vi "test - Basic Function.vi"(8 "error in (no error)":errorcluster, 11 "TestCase in":refnum<class "testcase-Broadcast Registry.lvclass">) -> (0 "error out":errorcluster, 3 "TestCase out":refnum<class "testcase-Broadcast Registry.lvclass">)   [LabVIEW 2017, in "testcase-Broadcast Registry.lvclass"]
uses:
  testcase-Broadcast Registry.lvclass
  f1ab6f25-c30d-499f-96ca-3a55fa643449.vi
  src/user.lib/_NEVSTOP/Communicable State Machine(CSM)/AdvanceAPI/CSM - Revert Arguments-Safe String.vi
  src/user.lib/_NEVSTOP/Communicable State Machine(CSM)/_Shared/Trim Single-line Text.vi
  src/user.lib/_NEVSTOP/Communicable State Machine(CSM)/AdvanceAPI/CSM - Make String Arguments Safe.vi
  src/user.lib/_NEVSTOP/Communicable State Machine(CSM)/AdvanceAPI/CSM - Break Down Multiple States String.vi
  src/user.lib/_NEVSTOP/Communicable State Machine(CSM)/AdvanceAPI/CSM - Compact Multiple States.vi
  src/user.lib/_NEVSTOP/Communicable State Machine(CSM)/AdvanceAPI/CSM - Keywords.vi
  <vilib>/addons/_JKI Toolkits/VI Tester/TestCase.llb/TestCase.lvclass
  src/user.lib/_NEVSTOP/Communicable State Machine(CSM)/Communicable State Machine.lvlib
  C:/Program Files (x86)/National Instruments/LabVIEW 2017/vi.lib/addons/_JKI Toolkits/VI Tester/TestCase.llb/TestCase.lvclass
panel:
  out "Error Occurred":errorcluster
  out "State History":string
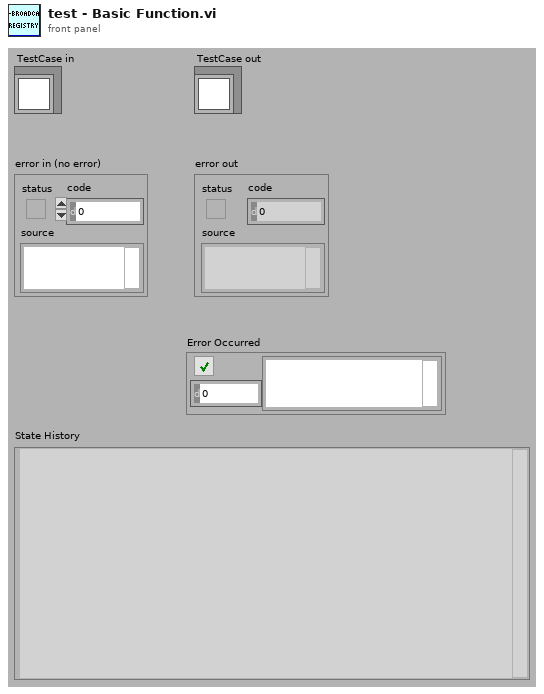
[diagram p1: front panel]
types:
  T1 = enum32{"Invalid", "Standard", "Closed", "Hidden", "Minimized", "Maximized"}
  T2 = enum32{"invalid app kind", "Development System", "Run Time System", "Student Edition", "Embedded LabVIEW", "Evaluation", "Custom"}
  T3 = cluster{"Status":string, "Source CSM":string, "Target CSM":string, "Target API":string}[]
  T4 = typedef "Communicable State Machine.lvlib/_CSM_Response Source Message.ctl" = cluster{"‘State":string, "’Arguments":string, "’Error":errorcluster}
  T5 = cluster{"Current VI Reference":refnum<vi>, "Close Panel on Exit?":bool}
  T6 = cluster{"Core":cluster{"Current VI Reference":refnum<vi>, "Close Panel on Exit?":bool}, "Your Boolean data":bool, "Your string data":string}
  T7 = cluster{"Status":string, "Source CSM":string, "Target CSM":string, "Target API":string}
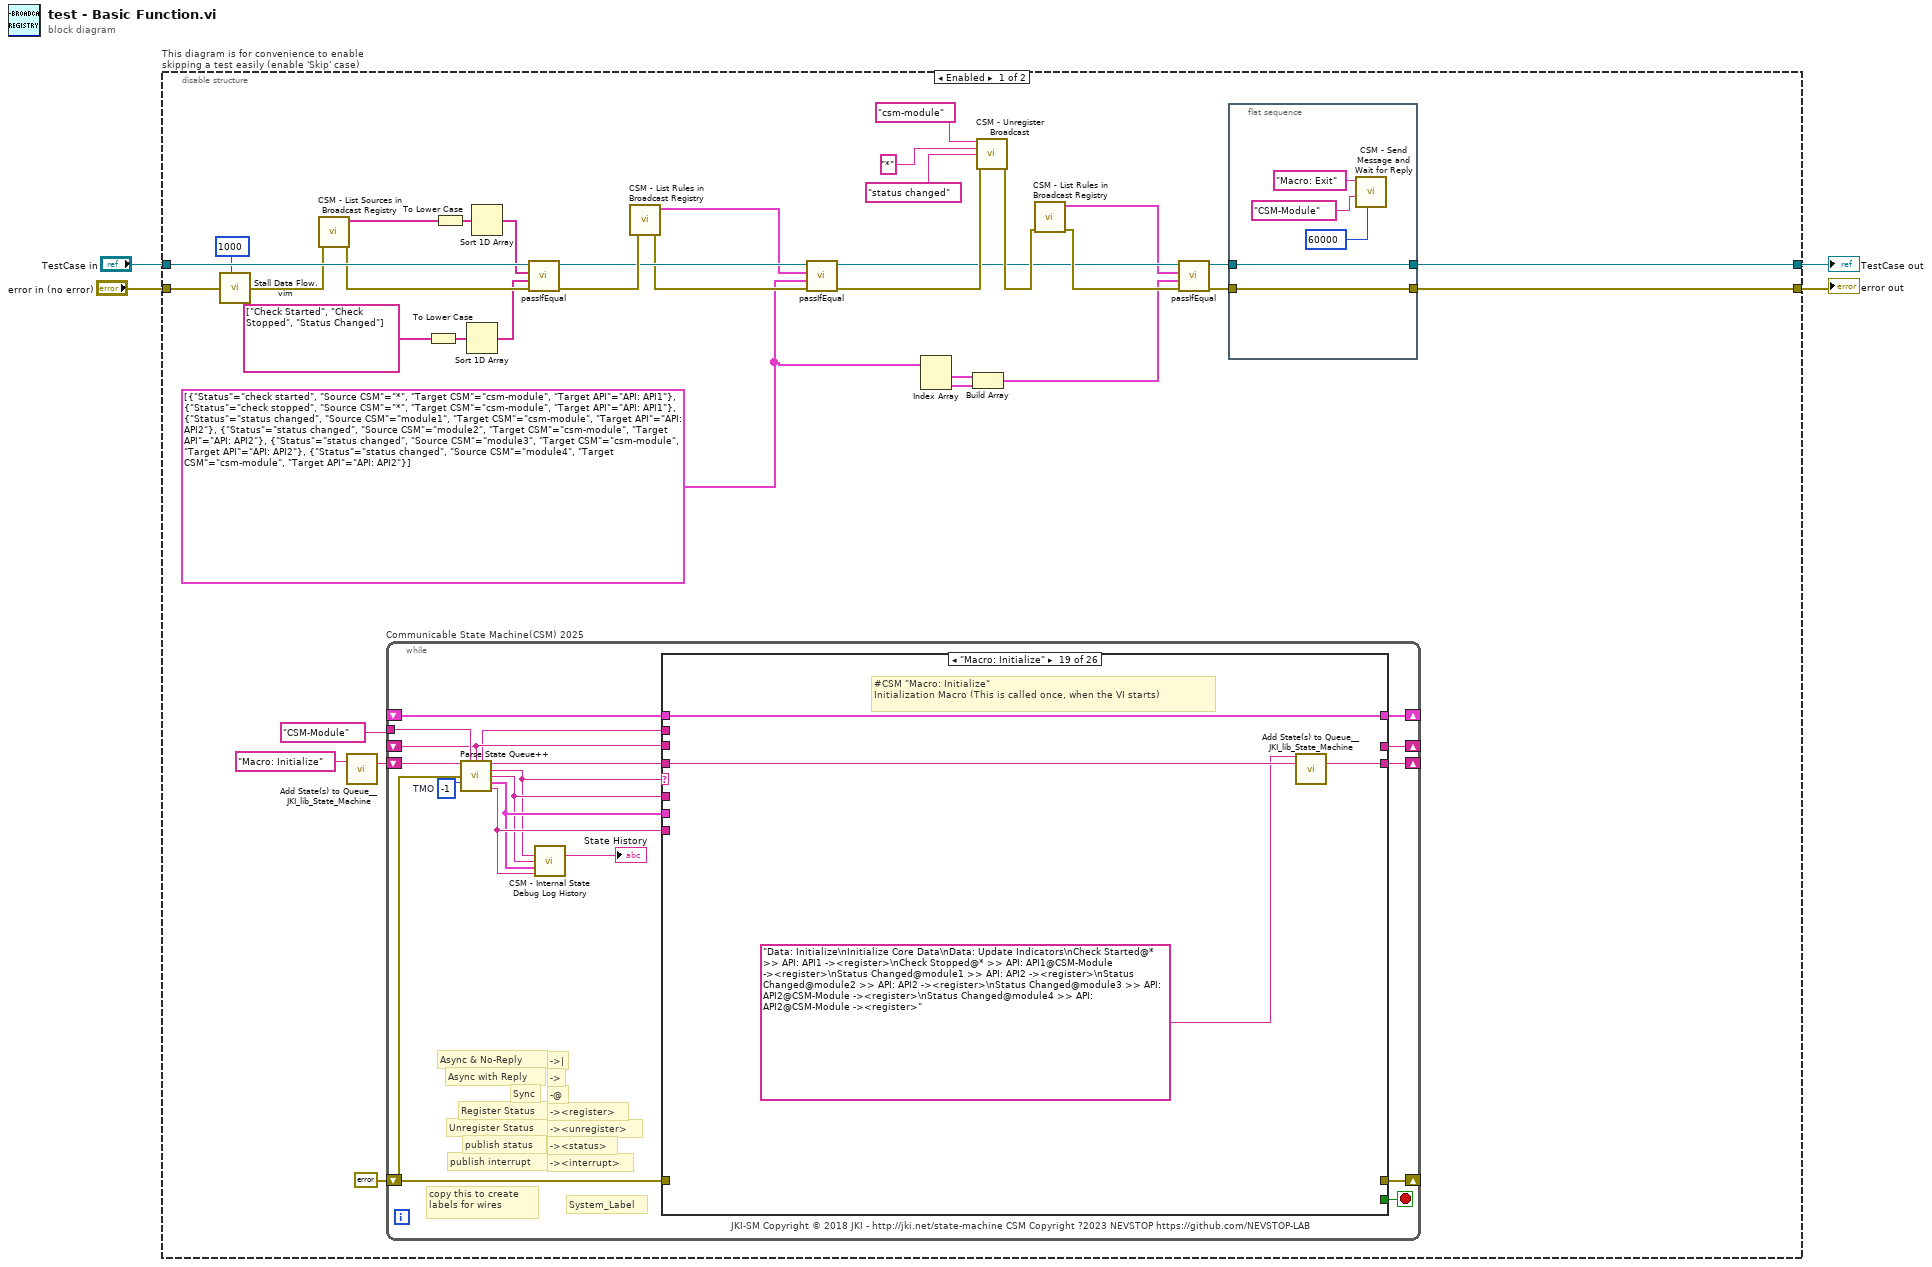
[diagram p0: block diagram]
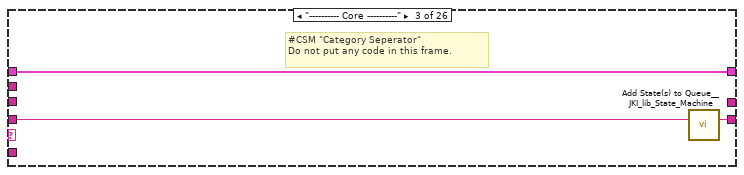
[diagram p4: hidden frame]
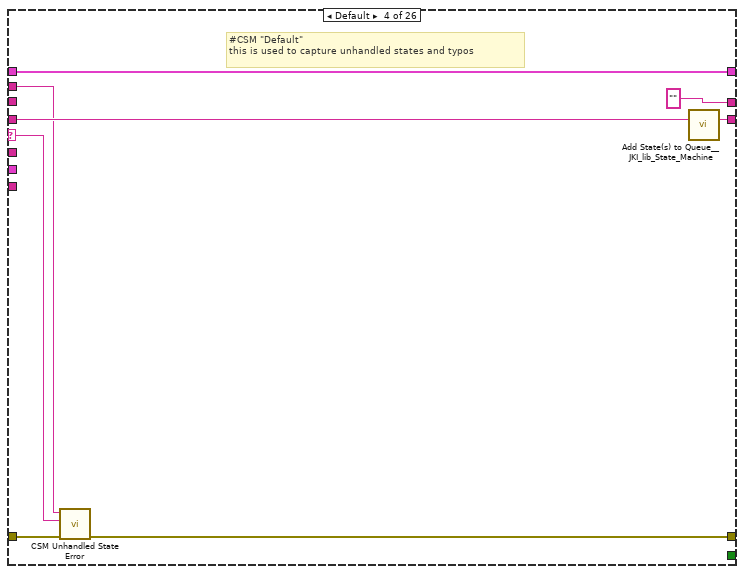
[diagram p5: hidden frame]
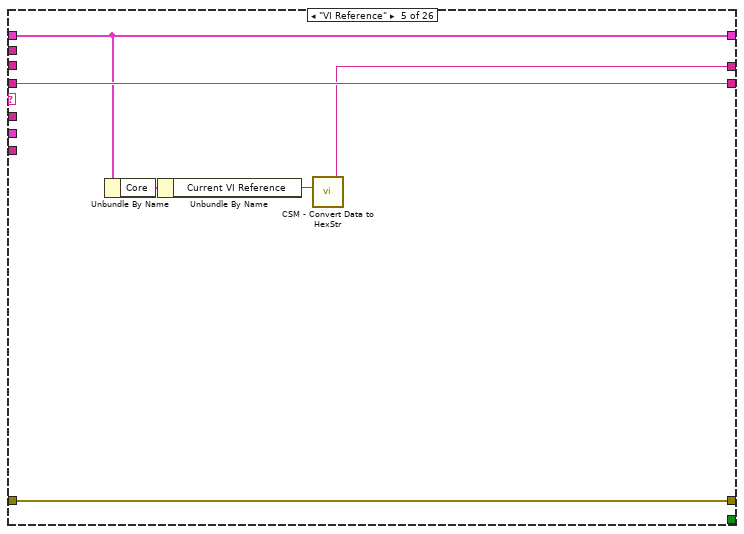
[diagram p6: hidden frame]
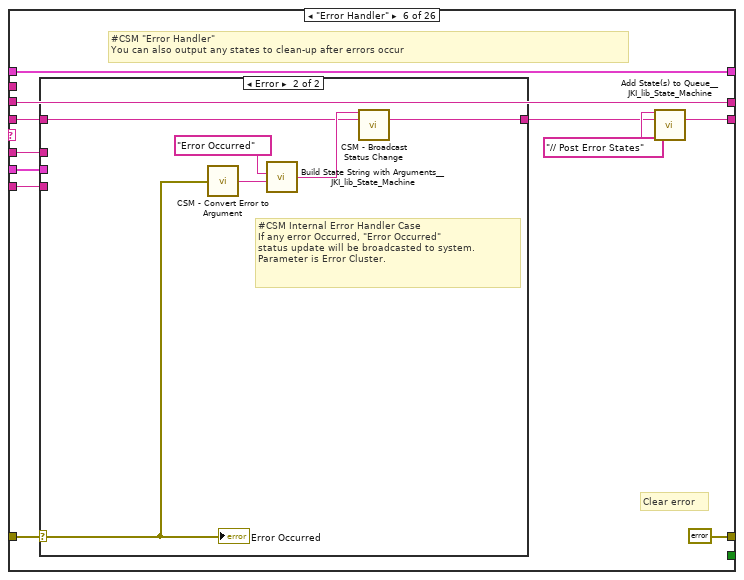
[diagram p7: hidden frame]
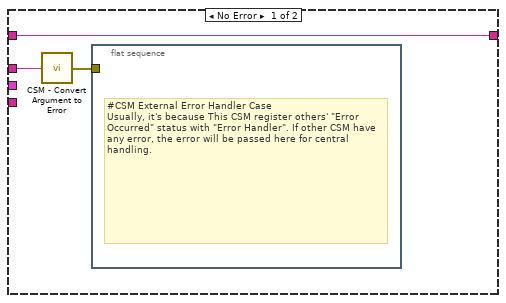
[diagram p8: hidden frame]
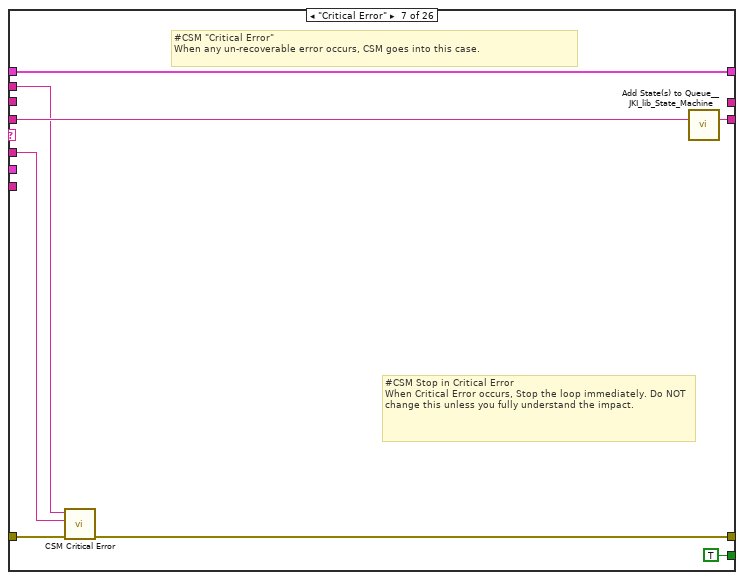
[diagram p9: hidden frame]
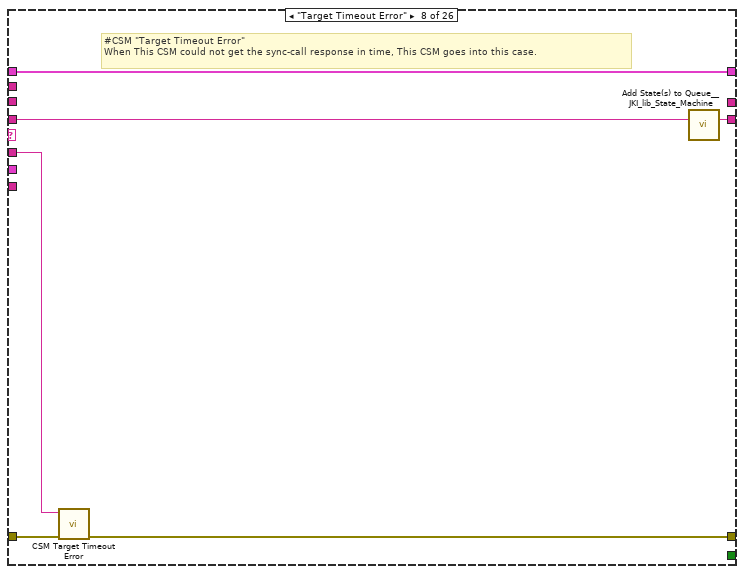
[diagram p10: hidden frame]
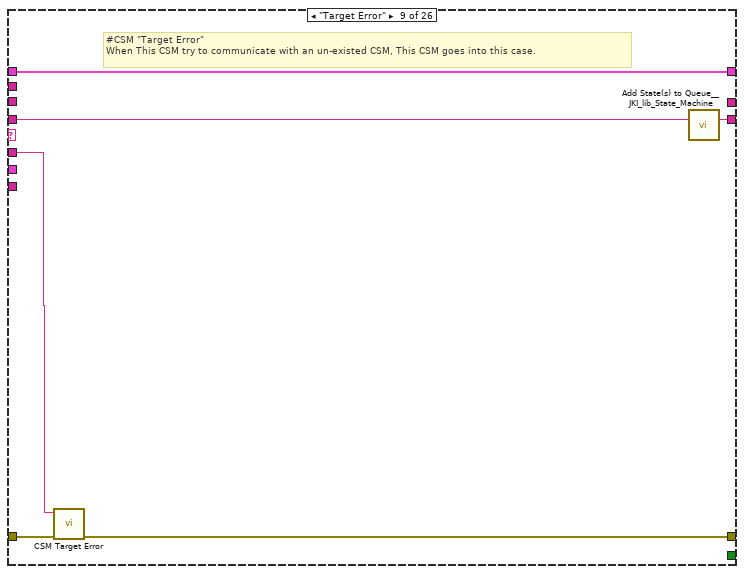
[diagram p11: hidden frame]
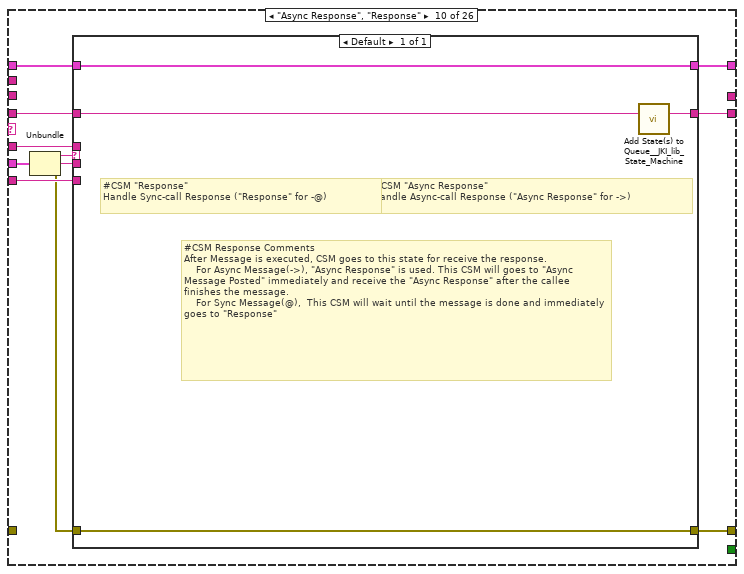
[diagram p12: hidden frame]
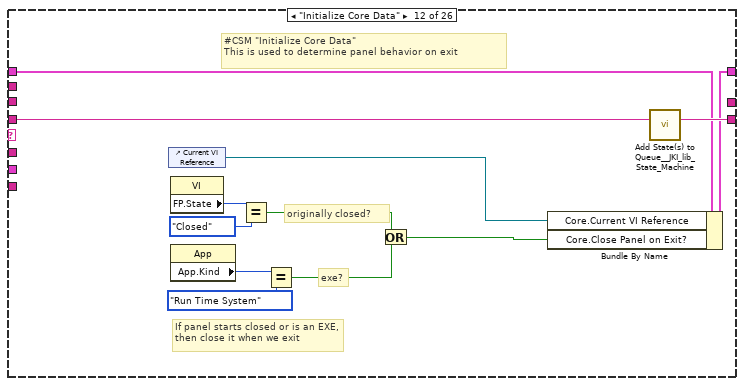
[diagram p14: hidden frame]
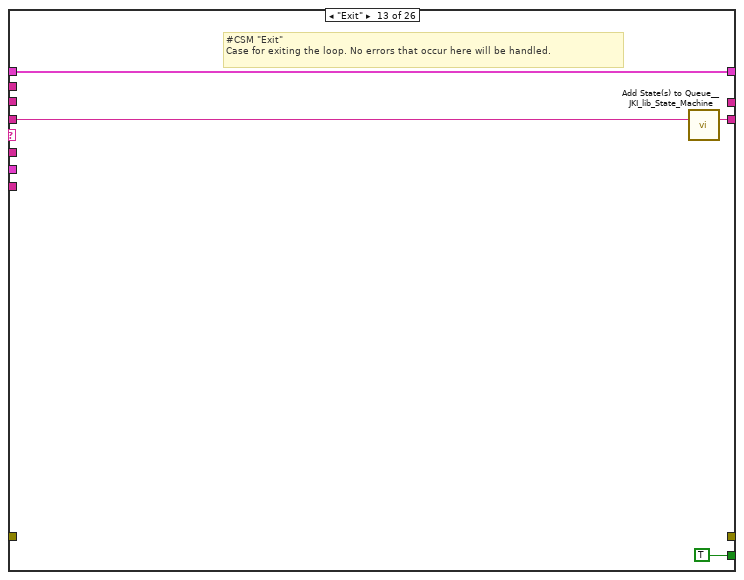
[diagram p15: hidden frame]
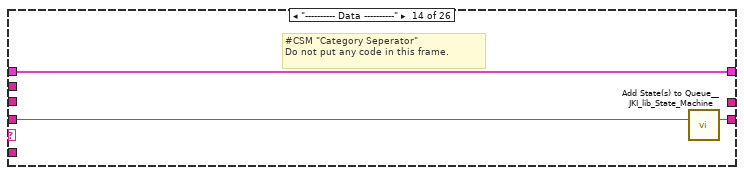
[diagram p16: hidden frame]
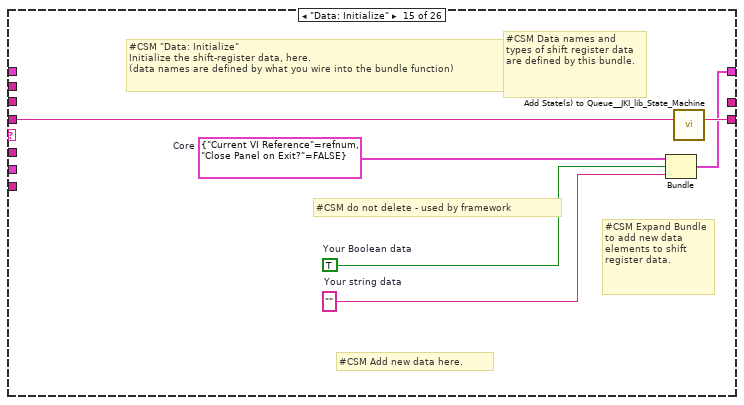
[diagram p17: hidden frame]
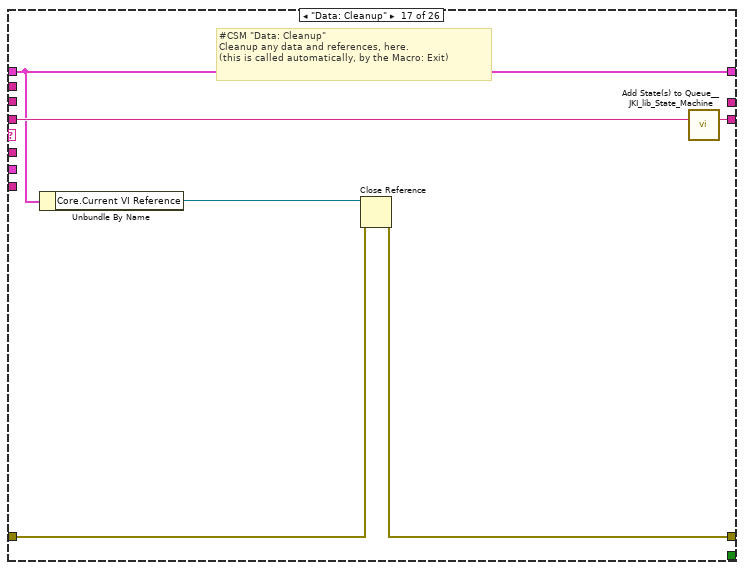
[diagram p19: hidden frame]
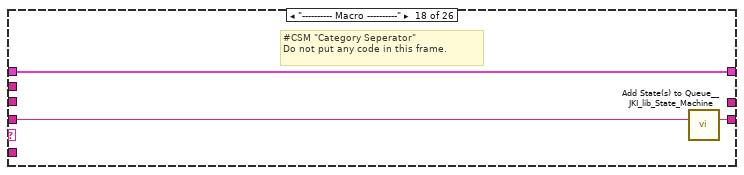
[diagram p20: hidden frame]
diagram:
  n1 = disable-structure "This diagram is for convenience to enable skipping a test easily (enable 'Skip' case)" shown="Enabled" {
    disable-tunnel: "TestCase in" -> [w39 w210]
    disable-tunnel: [w21 w208] -> w1
    disable-tunnel: [w28 w209] -> w3
    disable-tunnel: "error in (no error)" -> [w38 w207]
    frame Enabled {
      w8 = T3 [{"Status"="check started", "Source CSM"="*", "Target CSM"="csm-module", "Target API"="API: API1"}, {"Status"="check stopped", "Source CSM"="*", "Target CSM"="csm-module", "Target API"="API: API1"}, {"Status"="status changed", "Source CSM"="module1", "Target CSM"="csm-module", "Target API"="API: API2"}, {"Status"="status changed", "Source CSM"="module2", "Target CSM"="csm-module", "Target API"="API: API2"}, {"Status"="status changed", "Source CSM"="module3", "Target CSM"="csm-module", "Target API"="API: API2"}, {"Status"="status changed", "Source CSM"="module4", "Target CSM"="csm-module", "Target API"="API: API2"}] ("Entries")
      n2 = call "Stall Data Flow.vim"("value in"=w38, "milliseconds to wait"=u32 1000) -> ("value out"=w33:errorcluster)  [unwired: 1 out]
      n3 = call "CSM - List Sources in Broadcast Registry.vi"("error in (no error)"=w33) -> ("error out"=w31:errorcluster, "Broadcast Names"=w30:string[])  [unwired: 9 in]
      n4 = call <vilib>:"Add State(s) to Queue__JKI_lib_State_Machine.vi"("State(s) in (\"\")"="Macro: Initialize" ("Init State(\"Macro: Initialize\")")) -> ("States Out"=w37:string)  [unwired: 14 in]
      n5 = while "Communicable State Machine(CSM) 2025" {
        shift-right: [w57] -> _
        shift-left: _ -> [w56]
        shift-right: [w60] -> _
        shift-left: errorcluster {"status"=FALSE, "code"=0, "source"=""} ("error out") -> [w46]
        shift-right: [w59] -> _
        shift-left: w37 -> [w61]
        tunnel: "CSM-Module" ("Name (\"\" to Use UUID)") -> [w53]
        shift-right: [w54] -> _
        shift-left: _ -> [w48]
        stop <- w58 stop-if-true
        w55 = -1  # TMO
        # "-><interrupt>"
        # "-><status>"
        # "-><unregister>"
        # "-><register>"
        # "-@"
        # "->"
        # "->|"
        # "publish interrupt"
        # "publish status"
        # "Unregister Status"
        # "Register Status"
        # "Sync"
        # "Async with Reply"
        # "Async & No-Reply"
        # "JKI-SM Copyright © 2018 JKI - http://jki.net/state-machine CSM Copyright ?2023 NEVSTOP https://github.com/NEVSTOP-LAB"
        # "copy this to create labels for wires"
        # "System_Label"
        n6 = call "Parse State Queue++.vi"("State Queue"=w61, "Name (\"\" to Use UUID)"=w53, "Response Arguments"=w48, "Previous Error"=w46, "Dequeue (1 ms)"=w55) -> ("Name Used"=w47:string, "Remaining States"=w62:string, "Current State"=w49:string, "Arguments"=w50:string, "Additional Information"=w51:T4, "Source CSM"=w52:string)  [unwired: 5 in]
        n7 = call "CSM - Internal State Debug Log History.vi"("State"=w49, "Arguments (\"\")"=w50, ">> Response Source Message >>"=w51, "Source (\"\")"=w52) -> ("Debug Log"=→"State History":string)  [unwired: 11 in]
        n8 = case shown="\"Macro: Initialize\"" w49 {
          selector: w49 -> [_ _ _ w73 _ _ _ _ _ _ _ _ _ _ _ _ _ _ _ _ _ _ _ _ _ _]
          tunnel: w62 -> [w63 w66 w69 w77 w82 w88 w111 w117 w123 w133 w140 w152 w156 w159 w165 w167 w173 w176 w180 w186 w188 w191 w195 w200 w203 w206]
          tunnel: w50 -> [_ _ _ _ _ w87 w107 w114 w120 w127 _ _ _ _ _ _ _ _ _ _ _ _ w193 _ _ _]
          tunnel: w56 -> [w64 w65 w67 w75 w81 w93 w109 w115 w121 w131 w139 w146 w154 w157 _ w166 w168 w174 w178 w184 w187 w190 w194 w198 w201 w204]
          tunnel: [_ _ _ w70 w83 errorcluster {"status"=FALSE, "code"=0, "source"=""} ("error out") w104 w112 w118 w134 _ _ _ _ _ _ w169 _ _ _ _ _ _ _ _ _] -> w60
          tunnel: w46 -> [_ _ _ w71 w83 w91 w105 w113 w119 _ _ _ _ _ _ _ w170 _ _ _ _ _ _ _ _ _]
          tunnel: [w63 w66 w68 w76 w82 w89 w110 w116 w122 w132 w140 w151 w155 w158 w164 w167 w172 w175 w179 w185 w188 w191 w195 w199 w202 w205] -> w59
          tunnel: [_ _ _ _ _ _ TRUE _ _ _ _ _ TRUE _ _ _ _ _ _ _ _ _ _ _ _ _] -> w58
          tunnel: [w64 w65 w67 w75 w81 w93 w109 w115 w121 w130 w139 w150 w154 w157 w163 w166 w168 w174 w178 w184 w187 w190 w194 w198 w201 w204] -> w57
          tunnel: w52 -> [_ _ _ _ _ w86 _ _ _ w128 _ _ _ _ _ _ _ _ _ _ _ _ _ _ _ _]
          tunnel: w51 -> [_ _ _ _ _ w85 _ _ _ w129 _ _ _ _ _ _ _ _ _ _ _ _ _ _ _ _]
          tunnel: [_ _ _ "" w78 w84 _ _ _ _ _ _ _ _ _ _ _ _ _ _ _ "API1 Response" w192 _ _ _] -> w54
          tunnel: w47 -> [_ _ _ w72 _ _ w106 _ _ _ _ _ _ _ _ _ _ _ _ _ _ _ _ _ _ _]
          tunnel: w48 -> [_ _ _ _ _ w84 _ _ _ _ _ _ _ _ _ _ _ _ _ _ _ _ _ _ _ _]
          frame "", "Idle" {
            # "#CSM \"Idle/Event Handler\"\nexecutes when the state queue is empty"
          }
          frame "CSM Documentation" {
            # "#CSM Documentation"
            # "#CSM State Syntax\n\n// Comment line, all text to the right of “//” will be ignored\n// Local Message Example\nDoSth: DoA >> Arguments\n\n// Sync Call Example\nAPI: xxxx >> Arguments -@ TargetModule\n\n// Async Call Example\nAPI: xxxx >> Arguments -> TargetModule\n\n// Async Call without Reply Example\nAPI: xxxx >> Arguments ->| TargetModule\n\n// Broadcast normal status:\nStatus >> StatusArguments  -><status>\n\n// Broadcast Interrupt status:\nInterrupt >> StatusArguments  -><interrupt>\n\n// Register Source Module's status to Handler Module\nStatus@Source Module >> Handler Module@Handler Module -><register>\n\n// Unegister Source Module's status\nStatus@Source Module >> Handler Module -><unregister>"
            # "#CSM README FIRST\n\nCommunicable State Machine(CSM) is a LabVIEW application framework that builds upon JKI State Machine(JKISM). It follows the pattern of JKISM and extends the keywords to describe message communication between modules, including concepts such as Sync-Message, Async-Message, Subscription/Unsubscription of status - essential elements for creating reusable code modules. For more information, please visit the CSM wiki: https://nevstop-lab.github.io/CSM-Wiki/\n\nFor instructions on JKI State Machine, visit: \n    http://jki.net/state-machine/\nFor information about CSM, visit: \n    https://github.com/NEVSTOP-LAB"
            # "#CSM \"Documentation\"\nCase for holding CSM Documenation"
          }
          frame "---------- Core ----------" {
            # "#CSM \"Category Seperator\"\nDo not put any code in this frame."
            n9 = call <vilib>:"Add State(s) to Queue__JKI_lib_State_Machine.vi"("State(s) in (\"\")"=w69) -> ("States Out"=w68:string)  [unwired: 14 in]
          }
          frame Default {
            # "#CSM \"Default\"\nthis is used to capture unhandled states and typos"
            n10 = call "CSM Unhandled State Error.vi"("error in (no error)"=w71, "Undefined State"=w73, "CSM Name"=w72) -> ("error out"=w70:errorcluster)  [unwired: 8 in]
            n11 = call <vilib>:"Add State(s) to Queue__JKI_lib_State_Machine.vi"("State(s) in (\"\")"=w77) -> ("States Out"=w76:string)  [unwired: 14 in]
          }
          frame "VI Reference" {
            n12 = Unbundle By Name(w81) -> ("Core"=w80:T5)
            n13 = Unbundle By Name(w80) -> ("Current VI Reference"=w79:refnum<vi>)
            n14 = call "CSM - Convert Data to HexStr.vi"("Variant"=w79) -> ("HEX String (0-9,A-F)"=w78:string)  [unwired: 8 in]
          }
          frame "Error Handler" {
            # "#CSM \"Error Handler\"\nYou can also output any states to clean-up after errors occur"
            # "Clear error"
            n15 = case shown="Error" w91 {
              selector: w91 -> [_ w98]
              tunnel: [w97 w100] -> w90
              tunnel: w88 -> [w97 w99]
              tunnel: w87 -> [w96 _]
              tunnel: w86 -> [_ _]
              tunnel: w85 -> [_ _]
              frame No Error {
                n16 = call "CSM - Convert Argument to Error.vi"("Argument"=w96) -> ("Error"=w95:errorcluster)  [unwired: 4 in]
                n17 = flat-sequence {
                  tunnel: w95 -> [_]
                  frame #0 {
                    # "#CSM External Error Handler Case\nUsually, it's because This CSM register others' \"Error Occurred\" status with \"Error Handler\". If other CSM have any error, the error will be passed here for central handling."
                  }
                }
              }
              frame Error {
                # "#CSM Internal Error Handler Case \nIf any error Occurred, \"Error Occurred\" \nstatus update will be broadcasted to system.\nParameter is Error Cluster."
                n18 = call "CSM - Convert Error to Argument.vi"("Error"=w98) -> ("Argument"=w102:string)  [unwired: 4 in]
                n19 = call <vilib>:"Build State String with Arguments__JKI_lib_State_Machine.vi"("Arguments (\"\")"=w102, "State"="Error Occurred" ("Status with Arguments")) -> ("State with Arguments"=w101:string)  [unwired: 4 in]
                n20 = call "CSM - Broadcast Status Change.vi"("Status With Arguments"=w101, "State Queue"=w99) -> ("Remaining States"=w100:string)  [unwired: 13 in]
                "Error Occurred" <- w98
              }
            }
            n21 = call <vilib>:"Add State(s) to Queue__JKI_lib_State_Machine.vi"("State(s) in Front (\"\")"="// Post Error States", "State(s) in (\"\")"=w90) -> ("States Out"=w89:string)  [unwired: 13 in]
          }
          frame "Critical Error" {
            # "#CSM \"Critical Error\"\nWhen any un-recoverable error occurs, CSM goes into this case."
            # "#CSM Stop in Critical Error\nWhen Critical Error occurs, Stop the loop immediately. Do NOT change this unless you fully understand the impact."
            n22 = call "CSM Critical Error.vi"("error in (no error)"=w105, "Arugments (As Reason)"=w107, "CSM Name"=w106) -> ("error out"=w104:errorcluster)  [unwired: 8 in]
            n23 = call <vilib>:"Add State(s) to Queue__JKI_lib_State_Machine.vi"("State(s) in (\"\")"=w111) -> ("States Out"=w110:string)  [unwired: 14 in]
          }
          frame "Target Timeout Error" {
            # "#CSM \"Target Timeout Error\"\nWhen This CSM could not get the sync-call response in time, This CSM goes into this case."
            n24 = call "CSM Target Timeout Error.vi"("error in (no error)"=w113, "Arguments (As CSM Name)"=w114) -> ("error out"=w112:errorcluster)  [unwired: 9 in]
            n25 = call <vilib>:"Add State(s) to Queue__JKI_lib_State_Machine.vi"("State(s) in (\"\")"=w117) -> ("States Out"=w116:string)  [unwired: 14 in]
          }
          frame "Target Error" {
            # "#CSM \"Target Error\"\nWhen This CSM try to communicate with an un-existed CSM, This CSM goes into this case."
            n26 = call "CSM Target Error.vi"("error in (no error)"=w119, "Arguments (As CSM Name)"=w120) -> ("error out"=w118:errorcluster)  [unwired: 9 in]
            n27 = call <vilib>:"Add State(s) to Queue__JKI_lib_State_Machine.vi"("State(s) in (\"\")"=w123) -> ("States Out"=w122:string)  [unwired: 14 in]
          }
          frame "Async Response", "Response" {
            n28 = Unbundle(w129) -> ("‘State"=w126:string, "’Arguments"=w125:string, "’Error"=w124:errorcluster)
            n29 = case shown="Default" w126 {
              tunnel: [w135] -> w132
              tunnel: w133 -> [w136]
              tunnel: [w138] -> w130
              tunnel: w131 -> [w138]
              tunnel: [w137] -> w134
              tunnel: w124 -> [w137]
              tunnel: w128 -> [_]
              tunnel: w127 -> [_]
              tunnel: w125 -> [_]
              frame Default {
                # "#CSM \"Async Response\"\nHandle Async-call Response (\"Async Response\" for ->)"
                # "#CSM \"Response\"\nHandle Sync-call Response (\"Response\" for -@)"
                # "#CSM Response Comments\nAfter Message is executed, CSM goes to this state for receive the response.\n    For Async Message(->), \"Async Response\" is used. This CSM will goes to \"Async Message Posted\" immediately and receive the \"Async Response\" after the callee finishes the message.\n    For Sync Message(@),  This CSM will wait until the message is done and immediately goes to \"Response\""
                n30 = call <vilib>:"Add State(s) to Queue__JKI_lib_State_Machine.vi"("State(s) in (\"\")"=w136) -> ("States Out"=w135:string)  [unwired: 14 in]
              }
            }
          }
          frame "Async Message Posted" {
            # "#CSM \"Async Message Posted\"\nAfter Async Message is posted (-> or ->| ), CSM goes to this state for post-action.\nYou can use Argument - State to tell which Async Message is called."
          }
          frame "Initialize Core Data" {
            # "#CSM \"Initialize Core Data\"\nThis is used to determine panel behavior on exit"
            # "originally closed?"
            # "exe?"
            # "If panel starts closed or is an EXE, then close it when we exit"
            n31 = control-ref of="Current VI Reference"() -> (w144:refnum<vi>)
            n32 = property class="VI"() -> ("FP.State"=w143:T1)  [unwired: 2 in, 2 out]
            n33 = property class="App"() -> ("App.Kind"=w149:T2)  [unwired: 2 in, 2 out]
            n34 = Equal?(x=w143, y=T1."Closed" ("Front Panel Window:State")) -> (x = y?=w141:bool)
            n35 = Equal?(x=w149, y=T2."Run Time System" ("Application:Kind")) -> (x = y?=w147:bool)
            n36 = Or(x=w141, y=w147) -> (x .or. y?=w145:bool)
            n37 = Bundle By Name(cluster=w146, "Core.Current VI Reference"=w144, "Core.Close Panel on Exit?"=w145) -> (w150:T6)
            n38 = call <vilib>:"Add State(s) to Queue__JKI_lib_State_Machine.vi"("State(s) in (\"\")"=w152) -> ("States Out"=w151:string)  [unwired: 14 in]
          }
          frame "Exit" {
            # "#CSM \"Exit\"\nCase for exiting the loop. No errors that occur here will be handled."
            n39 = call <vilib>:"Add State(s) to Queue__JKI_lib_State_Machine.vi"("State(s) in (\"\")"=w156) -> ("States Out"=w155:string)  [unwired: 14 in]
          }
          frame "---------- Data ----------" {
            # "#CSM \"Category Seperator\"\nDo not put any code in this frame."
            n40 = call <vilib>:"Add State(s) to Queue__JKI_lib_State_Machine.vi"("State(s) in (\"\")"=w159) -> ("States Out"=w158:string)  [unwired: 14 in]
          }
          frame "Data: Initialize" {
            w160 = T5 {"Current VI Reference"=refnum, "Close Panel on Exit?"=FALSE}  # Core
            w162 = TRUE  # Your Boolean data
            w161 = ""  # Your string data
            # "#CSM \"Data: Initialize\"\nInitialize the shift-register data, here.\n(data names are defined by what you wire into the bundle function)"
            # "#CSM do not delete - used by framework"
            # "#CSM Expand Bundle to add new data elements to shift register data."
            # "#CSM Add new data here."
            # "#CSM Data names and types of shift register data are defined by this bundle."
            n41 = Bundle("Core"=w160, "Your Boolean data"=w162, "Your string data"=w161) -> (w163:T6)  [unwired: 1 in]
            n42 = call <vilib>:"Add State(s) to Queue__JKI_lib_State_Machine.vi"("State(s) in (\"\")"=w165) -> ("States Out"=w164:string)  [unwired: 14 in]
          }
          frame "Data: Update Indicators" {
          }
          frame "Data: Cleanup" {
            # "#CSM \"Data: Cleanup\"\nCleanup any data and references, here.\n(this is called automatically, by the Macro: Exit)"
            n43 = Unbundle By Name(w168) -> ("Core.Current VI Reference"=w171:refnum<vi>)
            n44 = Close Reference(reference=w171, error in (no error)=w170) -> (error out=w169:errorcluster)
            n45 = call <vilib>:"Add State(s) to Queue__JKI_lib_State_Machine.vi"("State(s) in (\"\")"=w173) -> ("States Out"=w172:string)  [unwired: 14 in]
          }
          frame "---------- Macro ----------" {
            # "#CSM \"Category Seperator\"\nDo not put any code in this frame."
            n46 = call <vilib>:"Add State(s) to Queue__JKI_lib_State_Machine.vi"("State(s) in (\"\")"=w176) -> ("States Out"=w175:string)  [unwired: 14 in]
          }
          frame "Macro: Initialize" {
            # "#CSM \"Macro: Initialize\"\nInitialization Macro (This is called once, when the VI starts)"
            n47 = call <vilib>:"Add State(s) to Queue__JKI_lib_State_Machine.vi"("State(s) in Front (\"\")"="Data: Initialize\nInitialize Core Data\nData: Update Indicators\nCheck Started@* >> API: API1 -><register>\nCheck Stopped@* >> API: API1@CSM-Module -><register>\nStatus Changed@module1 >> API: API2 -><register>\nStatus Changed@module2 >> API: API2 -><register>\nStatus Changed@module3 >> API: API2@CSM-Module -><register>\nStatus Changed@module4 >> API: API2@CSM-Module -><register>", "State(s) in (\"\")"=w180) -> ("States Out"=w179:string)  [unwired: 13 in]
          }
          frame "Macro: Exit" {
            # "#CSM \"Macro: Exit\"\nExit Macro (This is called once, when the VI exits)"
            n48 = call <vilib>:"Add State(s) to Queue__JKI_lib_State_Machine.vi"("State(s) in Front (\"\")"="//Exit Sub-Modules ", "State(s) at Back (\"\")"="Data: Cleanup\nExit") -> ("States Out"=w182:string)  [unwired: 13 in]
            n49 = call <vilib>:"Add State(s) to Queue__JKI_lib_State_Machine.vi"("State(s) in Front (\"\")"=w182, "State(s) in (\"\")"=w186) -> ("States Out"=w185:string)  [unwired: 13 in]
          }
          frame "---------- API ----------" {
            # "#CSM \"Category Seperator\"\nDo not put any code in this frame."
          }
          frame "API: API1" {
            # "#CSM API Example\nCopy/Rename this case for your own API"
            # "#CSM >> Msg/Rep's CSM >>\nIf you need to tell who triggered this state , use this string. If it's this case itself, this string is \"\"."
            # "#CSM >> Arguments >>\nDeal with the parameter if any"
            # "#CSM Response\nConnect this to return the response of your API"
          }
          frame "API: API2" {
            # "#CSM API Example\nCopy/Rename this case for your own API"
            # "unpack Hex String  to Variant\nif complex parameter is needed."
            n50 = call "CSM - Convert HexStr to Data.vi"("HEX String"=w193) -> ()  [unwired: 7 in, 2 out]
            n51 = disable-structure shown="Disabled" {
              disable-tunnel: [w196 "API2 Response"] -> w192
              frame Disabled {
                # "pack variant to hexstr \nif complex response is needed."
                # "complex Response"
                n52 = call "CSM - Convert Data to HexStr.vi"() -> ("HEX String (0-9,A-F)"=w196:string)  [unwired: 9 in]
              }
              frame Enabled {
              }
            }
          }
          frame "---------- Action ----------" {
            # "#CSM \"Category Seperator\"\nDo not put any code in this frame."
            n53 = call <vilib>:"Add State(s) to Queue__JKI_lib_State_Machine.vi"("State(s) in (\"\")"=w200) -> ("States Out"=w199:string)  [unwired: 14 in]
          }
          frame "Action: action1" {
            # "#CSM \"Internal State\"\nThis category is used for holding internal states"
            n54 = call <vilib>:"Add State(s) to Queue__JKI_lib_State_Machine.vi"("State(s) in (\"\")"=w203) -> ("States Out"=w202:string)  [unwired: 14 in]
          }
          frame "Action: action2" {
            # "#CSM \"Internal State\"\nThis category is used for holding internal states"
            n55 = call <vilib>:"Add State(s) to Queue__JKI_lib_State_Machine.vi"("State(s) in (\"\")"=w206) -> ("States Out"=w205:string)  [unwired: 14 in]
          }
        }
      }
      n56 = To Lower Case(string=string[] ["Check Started", "Check Stopped", "Status Changed"] ("Status in Registry")) -> (all lower case string=w25:string[])
      n57 = To Lower Case(string=w30) -> (all lower case string=w24:string[])
      n58 = Sort 1D Array(array=w25) -> (sorted array=w26:string[])
      n59 = Sort 1D Array(array=w24) -> (sorted array=w27:string[])
      n60 = call-dynamic "passIfEqual.vi"("error in (no error)"=w31, "y"=w26, "x"=w27, "TestCase in"=w39) -> ("error out"=w23:errorcluster, "TestCase out"=w22:refnum<class "testcase-Broadcast Registry.lvclass">)  [unwired: 6 in]
      n61 = call "CSM - List Rules in Broadcast Registry.vi"("error in (no error)"=w23) -> ("error out"=w20:errorcluster, "Rule Entries"=w18:T3)  [unwired: 8 in, 1 out]
      n62 = call-dynamic "passIfEqual.vi"("error in (no error)"=w20, "y"=w8, "x"=w18, "TestCase in"=w22) -> ("error out"=w19:errorcluster, "TestCase out"=w12:refnum<class "testcase-Broadcast Registry.lvclass">)  [unwired: 6 in]
      n63 = Index Array(array=w8) -> (element #1=w7:T7, element #2=w6:T7)  [unwired: 2 in]
      n64 = Build Array(w7, w6) -> (w5:T3)
      n65 = call "CSM - Unregister Broadcast.vi"("CSM Name(Empty for Broadcast Event)"="csm-module" ("CSM Name"), "Source CSM Name (* as Default)"="*", "Trigger"="status changed" ("Status"), "Error In"=w19) -> ("error out"=w14:errorcluster)  [unwired: 10 in, 1 out]
      n66 = call "CSM - List Rules in Broadcast Registry.vi"("error in (no error)"=w14) -> ("error out"=w13:errorcluster, "Rule Entries"=w9:T3)  [unwired: 8 in, 1 out]
      n67 = call-dynamic "passIfEqual.vi"("error in (no error)"=w13, "y"=w5, "x"=w9, "TestCase in"=w12) -> ("error out"=w10:errorcluster, "TestCase out"=w11:refnum<class "testcase-Broadcast Registry.lvclass">)  [unwired: 6 in]
      n68 = flat-sequence {
        tunnel: [w42] -> w28
        tunnel: w10 -> [w42]
        tunnel: [w41] -> w21
        tunnel: w11 -> [w41]
        frame #0 {
          n69 = call "CSM - Send Message and Wait for Reply.vi"("Response Timeout (-2 Using Global Settings)"=60000, "Target Module"="CSM-Module" ("Name (\"\" to Use UUID)"), "State"="Macro: Exit") -> ()  [unwired: 6 in, 3 out]
        }
      }
    }
    frame Disabled {
      # "skip test result while test is under development"
      n70 = call <vilib>:"skip.vi"("error in (no error)"=w207, "TestCase in"=w210) -> ("error out"=w209:errorcluster, "TestCase out"=w208:refnum<class "testcase-Broadcast Registry.lvclass">)  [unwired: 8 in]
    }
  }
  "error out" <- w3
  "TestCase out" <- w1
